vi "0x51_Read_description_one_table_parameter.vi"(8 "error in":errorcluster, 11 "paramUnicornIn in":T1) -> (0 "error out":errorcluster, 3 "paramUnicornIn out 2":T1)   [LabVIEW 2017, in "LV_Unicorn.lvlib"]
uses:
  LV_Unicorn.lvlib
  Control/unicorn_Param.ctl
  Control/unicorn_conn.ctl
  Control/unicorn_JSON.ctl
  Control/unicorn_ParamInt.ctl
  Control/unicorn_Telemetry.ctl
  Control/unicorn_Table.ctl
  Control/unicorn_ParamFloat.ctl
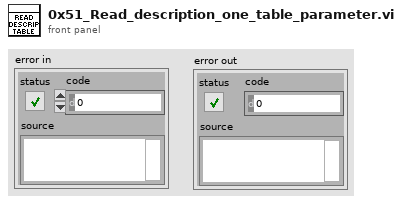
[diagram p1: front panel]
types:
  T1 = typedef "LV_Unicorn.lvlib/unicorn_Param.ctl" = cluster{"conParam":T2, "Param":T3}
  T2 = typedef "LV_Unicorn.lvlib/unicorn_conn.ctl" = cluster{"ReadIntParam":bool, "ReadDescrParam":bool, "ReadFloatParam":bool, "debug":bool, "ReadJSON":bool, "IP_address":string, "N_attempts":i32, "type_con":enum16{"Serial", "TCP"}, "MB_address":i32, "VISA":refnum<visa-resource-name>, "connection ID":refnum<k5>, "nameDevices":string, "timeout":i32, "port":u16, "type_version":string, "baud_rate":u32, "VersionControl":bool, "TCP_conn":bool, "WindowSize":i32}
  T3 = typedef "LV_Unicorn.lvlib/unicorn_JSON.ctl" = cluster{"NumParam":cluster{"NTelem":i32, "NInt":i32, "NFloat":i32, "NTable":i32}, "ParamInt":T4, "Telemetry":T5, "Table":T6, "ParamFloat":T7}
  T4 = typedef "LV_Unicorn.lvlib/unicorn_ParamInt.ctl" = cluster{"ID":string, "Num":i32, "Name":string, "Type":string, "Enum":string, "Desc":string, "Unit":string, "Access":string, "FormatStr":string, "Min":i32, "Max":i32}[]
  T5 = typedef "LV_Unicorn.lvlib/unicorn_Telemetry.ctl" = cluster{"ID":string, "Num":i32, "Name":string, "Desc":string, "Unit":string, "FormatStr":string, "Min":i32, "Max":i32}[]
  T6 = typedef "LV_Unicorn.lvlib/unicorn_Table.ctl" = cluster{"Num":i32, "Access":string, "ColumnCount":i32, "NeedParamPrepare":bool, "Columns":cluster{"Column":i32, "Desc":string, "Name":string}[], "DataType":string, "FormatStr":string, "ID":string, "Name":string, "RowCount":i32, "Rows":cluster{"Desc":string, "ID":string, "Max":i32, "Min":i32, "Name":string, "Row":i32, "Unit":string}[], "Type":string}[]
  T7 = typedef "LV_Unicorn.lvlib/unicorn_ParamFloat.ctl" = cluster{"ID":string, "Num":i32, "Name":string, "Type":string, "Enum":string, "Desc":string, "Unit":string, "Access":string, "FormatStr":string, "Min":sgl, "Max":sgl}[]
  T8 = cluster{"Num":i32, "Access":string, "ColumnCount":i32, "NeedParamPrepare":bool, "Columns":cluster{"Column":i32, "Desc":string, "Name":string}[], "DataType":string, "FormatStr":string, "ID":string, "Name":string, "RowCount":i32, "Rows":cluster{"Desc":string, "ID":string, "Max":i32, "Min":i32, "Name":string, "Row":i32, "Unit":string}[], "Type":string}
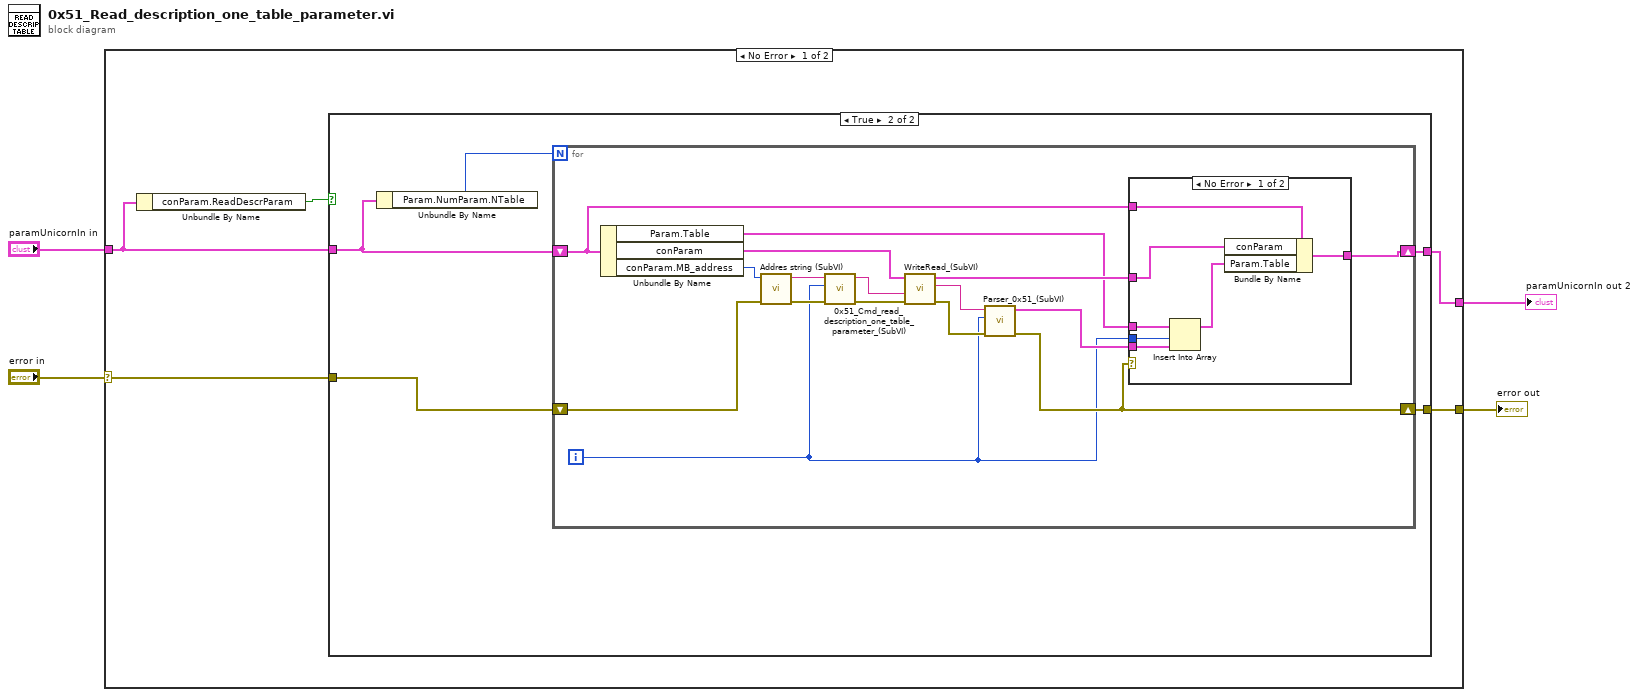
[diagram p0: block diagram]
diagram:
  n1 = case shown="No Error" "error in" {
    selector: "error in" -> [w9 w40]
    tunnel: [w7 w40] -> w4
    tunnel: "paramUnicornIn in" -> [w6 w39]
    tunnel: [w8 w39] -> w2
    frame No Error {
      n2 = Unbundle By Name(w6) -> ("conParam.ReadDescrParam"=w5:bool)
      n3 = case shown="True" w5 {
        tunnel: w9 -> [w10 w16]
        tunnel: [w11 w15] -> w8
        tunnel: [w10 w14] -> w7
        tunnel: w6 -> [w11 w12]
        frame False {
        }
        frame True {
          n4 = Unbundle By Name(w12) -> ("Param.NumParam.NTable"=w13:i32)
          n5 = for {
            N: w13 -> [_]
            shift-right: [w18] -> w14
            shift-left: w16 -> [w29]
            shift-right: [w28] -> w15
            shift-left: w12 -> [w20]
            i -> [w17]
            n6 = Unbundle By Name(w20) -> ("Param.Table"=w22:T6, "conParam"=w30:T2, "conParam.MB_address"=w26:i32)
            n7 = call "Addres string (SubVI).vi"("Адрес"=w26) -> ("String"=w25:string)  [unwired: 10 in]
            n8 = call "0x51_Cmd_read_description_one_table_parameter_(SubVI).vi"("NumberTableParam"=w17, "String in"=w25) -> ("String out"=w24:string)  [unwired: 9 in]
            n9 = call "WriteRead_(SubVI).vi"("error in"=w29, "Запрос"=w24, "ParamIn"=w30) -> ("error out"=w19:errorcluster, "Ответ"=w23:string, "ParamOut"=w27:T2)  [unwired: 4 in, 2 out]
            n10 = call "Parser_0x51_(SubVI).vi"("error in"=w19, "NumberTableParam"=w17, "String in"=w23) -> ("error out"=w18:errorcluster, "output cluster"=w21:T8)  [unwired: 6 in, 1 out]
            n11 = case shown="No Error" w18 {
              tunnel: [w37 w38] -> w28
              tunnel: w27 -> [w36 _]
              tunnel: w22 -> [w35 _]
              tunnel: w21 -> [w34 _]
              tunnel: w20 -> [w32 w38]
              tunnel: w17 -> [w31 _]
              frame No Error {
                n12 = Insert Into Array(array=w35, index=w31, new element=w34) -> (w33:T6)
                n13 = Bundle By Name(cluster=w32, "conParam"=w36, "Param.Table"=w33) -> (w37:T1)
              }
              frame Error {
              }
            }
          }
        }
      }
    }
    frame Error {
    }
  }
  "error out" <- w4
  "paramUnicornIn out 2" <- w2
